vi "TMP37.vi"(7 "Analog Ref Override":dbl, 8 "Error In":errorcluster, 10 "Analog Channel":u8, 11 "LINX Resource":T1) -> (0 "Error Out":errorcluster, 2 "Temp C":dbl, 3 "LINX Resource":T1)   [LabVIEW 2011, in "LVH-LINX.lvlib" / "TMP3x.lvlib"]
doc: "Read temperature from TMP37"
uses:
  TMP3x.lvlib
  Private/Type Defs/LINX Ref.ctl
  Private/Type Defs/Platform.ctl
  Private/Type Defs/Interface.ctl
  Private/Device/Type Defs/LINX Device Config.ctl
  Private/Device/Type Defs/TCP Config.ctl
  Private/Device/Type Defs/Channels.ctl
  Peripherals/Analog/Analog Read 1 Chan.vi
  LVH-LINX.lvlib
  Private/Device/Device.lvlib
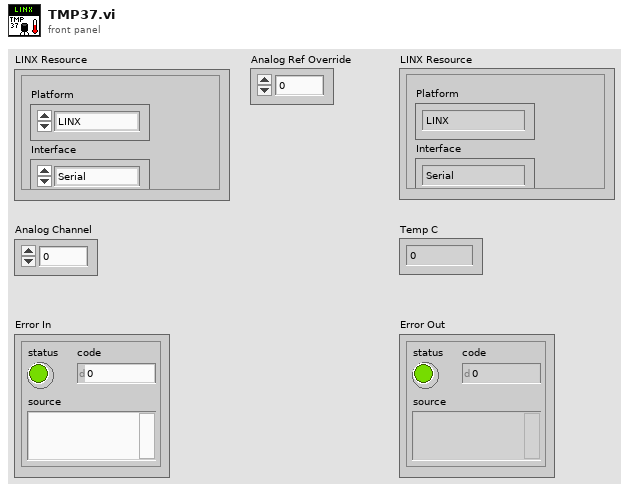
[diagram p1: front panel]
types:
  T1 = typedef "LVH-LINX.lvlib/LINX Ref.ctl" = cluster{"Platform":T2, "Interface":T3, "LINX Device Config":T4}
  T2 = typedef "LVH-LINX.lvlib/Platform.ctl" = enum16{"LINX", "myRIO"}
  T3 = typedef "LVH-LINX.lvlib/Interface.ctl" = enum16{"Serial", "TCP"}
  T4 = typedef "LVH-LINX.lvlib/Device.lvlib/LINX Device Config.ctl" = cluster{"Interface":T3, "COM Port":refnum<visa-resource-name>, "TCP Configuration":T5, "Device Family":u8, "Device ID":u8, "Device Name":string, "TCP Ref":refnum<k5>, "Channels":T6}
  T5 = typedef "LVH-LINX.lvlib/Device.lvlib/TCP Config.ctl" = cluster{"IP Address":string, "Port":u16}
  T6 = typedef "LVH-LINX.lvlib/Channels.ctl" = cluster{"DI":u8[], "DO":u8[], "AI":u8[], "AO":u8[], "PWM":u8[], "QE":u8[], "UART":u8[], "I2C 2":u8[], "SPI":u8[], "CAN":u8[], "Servo":u8[], "AI Ref (V)":dbl, "AO Ref (V)":dbl, "AO Resolution (Bits)":u8}
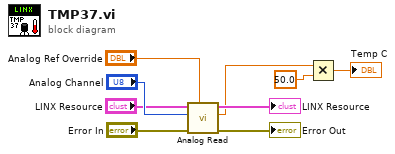
[diagram p0: block diagram]
diagram:
  n1 = call-poly "Analog Read.vi"("AI Range (V)"="Analog Ref Override", "Error In"="Error In", "Analog Channel"="Analog Channel", "LINX Resource"="LINX Resource") -> ("Error Out"=→"Error Out":errorcluster, "AI Value"=w3:dbl, "LINX Resource"=→"LINX Resource":T1)  [unwired: 4 in, 1 out]
  n2 = Multiply(x=w3, y=50.0) -> (x*y=→"Temp C":dbl)
